vi "2-4_Ch Gen 0-20mA Current_9265.vi"() -> ()   [LabVIEW 2010]
doc: "I. Description:\nThis example demonstrates how to generate a single current value on one or more current output channels.\n\nII. Instructions for Running:\n1. Select the physical channel or channels which correspond to where your signal is to be generated.\n2. Enter the minimum and maximum current ranges, in amps (not milliamps).\n3. Enter a current value to generate in the data array. There should be one array value for each channel specified in the Physical Channels control. The values will be generated in the order that they appear in the Physical Channels control. \nNote: Just like the minimum and maximum current ranges, the data values to generate are in units of amps, not milliamps. \n\nIII. Block Diagram Steps:\n1. Create an analog output current channel.\n2. Call the Start VI to start the task.\n3. Use the Write VI to generate the data values on the\nspecified channels. Each element in the array contains\none current value for one channel specified in the \nPhysical Channels control.\n4. Call the Clear Task VI to clear the Task.\n5. Return any errors to the user in a dialog box.\n\nIV. I/O Connections Overview:\nThe SCXI-1124 can operate on either an external or internal current source. The only difference is in the signal connections. When using the internal current source, connect a load between the SUPPLY and ISINK terminals. When using an external current source, connect the source and load to the ISINK and GND terminals. In either case, be sure that the channel numbers of the terminals used match the channel numbers specified in the Physical Channels control.\n\nNote: When using an external current source, be careful to avoid creating an uncontrolled current loop. See the SCXI-1124 User's Manual for more information. \n\nThe NI 6238 and NI 6239 devices require external current sources. See the M Series User Manual for more information about signal connections to these devices.\n\nThe output current can be measured by connecting an ammeter in series with the current loop. Alternatively, the current can be measured by replacing the load with a resistor of known value. By measuring the voltage across the resistor and dividing by the resistance, the current through the resistor can be calculated (Ohm's law)."
uses:
  <vilib>/Utility/error.llb/DialogType.ctl
  <vilib>/Platform/TimedLoop/XDataNode/XDataNode.xnode
  <vilib>/Platform/TimedLoop/XDataNode/timing_clust.ctl
  <vilib>/Platform/TimedLoop/XDataNode/nitl_modes.ctl
  <vilib>/Platform/TimedLoop/XDataNode/wakeup.ctl
  <vilib>/DAQmx/write.llb/DAQmx Write (Analog 1D DBL NChan 1Samp).vi
  <vilib>/DAQmx/create/channels.llb/DAQmx Create Channel (AO-Current-Basic).vi
  <vilib>/daqmx/miscellaneous.llb/DAQmx Fill In Error Info.vi
  <vilib>/Analysis/NI_AALBase.lvlib
  <vilib>/Platform/TimedLoop/XDataNode/XDNodeRunTimeDep.lvlib
panel:
  out "transposed array":dbl[][](array[numeric]) format="%.4f"
  in  "Sine?":bool
  in  "Continuous?":bool
  in  "Apply":bool
  in  "stop":bool
  in  "Physical Channels":tag="cDAQ1Mod7/ao0:1"
  in  "Data":dbl[](array[slide])=[0.0, 0.0] min=0.0 max=0.02 step=0.001 scale=0.0..0.02 scale format="%.3f"
  in  "Minimum Value":dbl format="%0.3f"
  in  "Maximum Value":dbl=0.02 format="%0.3f"
  # "For instructions, select Help>>Show Context Help"
  # "Channel Parameters"
  # "Change to: \nao0:3 for 4-Ch\nMode, and add\nto array below."
  # "Current Values"
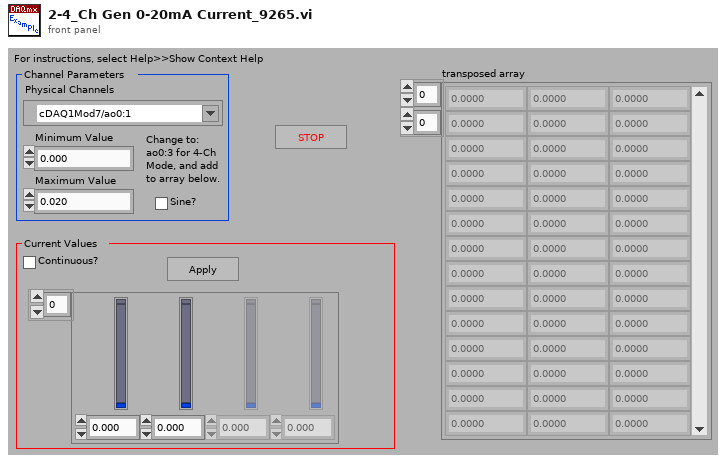
[diagram p1: front panel]
types:
  T1 = typedef "DialogType.ctl" = u16
  T2 = typedef "XDNodeRunTimeDep.lvlib/timing_clust.ctl" = cluster{"Expected End [f-1]":u64, "Actual End [f-1]":u64, "Finished Late? [f-1]":bool, "Expected End [i-1]":u64, "Actual End [i-1]":u64, "Finished Late? [i-1]":bool, "Expected Start [i]":u64, "Actual Start [i]":u64, "Expected Start [f]":u64, "Actual Start [f]":u64, "Source Name":string, "Structure Name":string, "Period":i64, "Deadline":i64, "Offset":i64, "Start":i64, "Priority":i32, "Timeout":i32, "Mode":T3, "Wakeup Reason":T4, "Error":errorcluster, "Source Type":string, "Secondary Source Type":string, "Global End Time":u64, "Global Start Time":u64, "Frame Duration":u64, "Iteration Duration":u64, "Assigned CPU":i32, "I/O Scan Engine Mode":u32}
  T3 = typedef "XDNodeRunTimeDep.lvlib/nitl_modes.ctl" = enum32{"No Change", "Process missed periods, maintain original phase", "Discard missed periods, maintain original phase", "Process missed periods, ignore original phase", "Discard missed periods, ignore original phase"}
  T4 = typedef "XDNodeRunTimeDep.lvlib/wakeup.ctl" = enum32{"Normal", "Aborted", "Asynchronous wakeup", "Timing source error", "Timed loop error", "Timeout"}
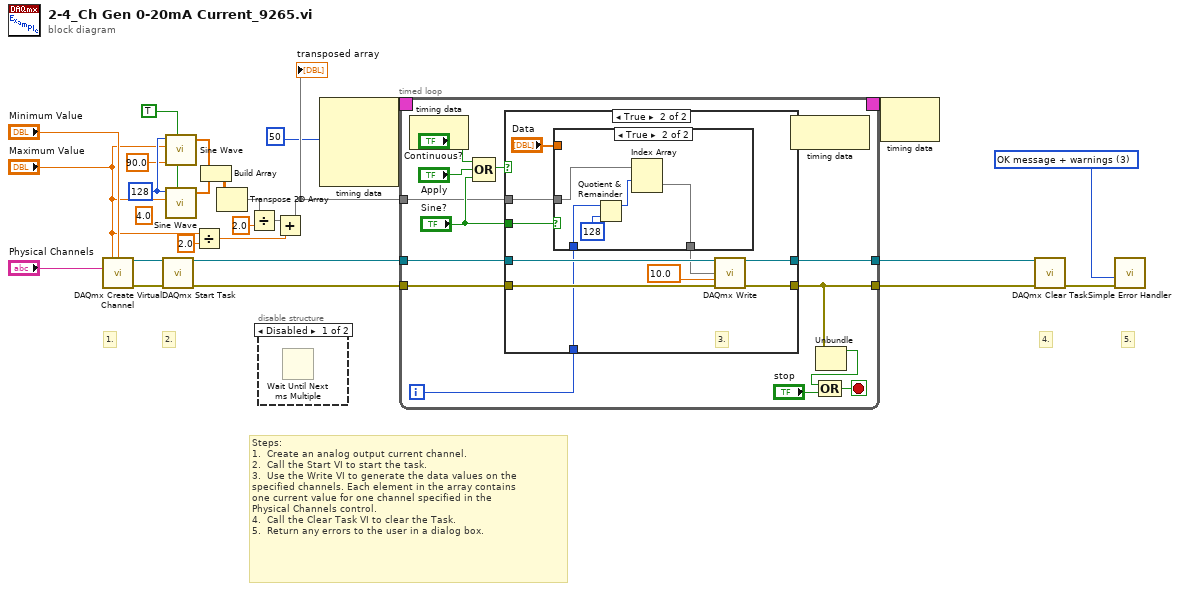
[diagram p0: block diagram]
diagram:
  w12 = TRUE ("reset phase")
  (unwired) 4.0 ("cycles")
  w16 = 128 ("samples")
  w19 = T1 3 items=["no dialog", "OK message", "continue or stop message", "OK message + warnings", "continue/stop + warnings"] ("type of dialog (OK msg:1)")
  # "5."
  # "Steps: \n1.  Create an analog output current channel.\n2.  Call the Start VI to start the task.\n3.  Use the Write VI to generate the data values on the\nspecified channels. Each element in the array contains\none current value for one channel specified in the \nPhysical Channels control.\n4.  Call the Clear Task VI to clear the Task.\n5.  Return any errors to the user in a dialog box."
  # "1."
  # "2."
  # "4."
  n1 = call-poly <vilib>:"DAQmx Create Virtual Channel.vi"("maximum value"="Maximum Value", "minimum value"="Minimum Value", "physical channels"="Physical Channels") -> ("task out"=w25:refnum<k21>, "error out"=w24:errorcluster)  [unwired: 11 in]
  n2 = call <vilib>:"DAQmx Start Task.vi"("task/channels in"=w25, "error in"=w24) -> ("task out"=w23:refnum<k21>, "error out"=w22:errorcluster)  [unwired: 12 in]
  n3 = call <vilib>:"Sine Wave.vi"("samples"=w16, "amplitude"="Maximum Value", "phase in"=90.0 ("phase(degrees)"), "reset phase"=w12) -> ("sine wave"=w15:dbl[])  [unwired: 1 in, 2 out]
  n4 = call <vilib>:"Sine Wave.vi"("samples"=w16, "amplitude"="Maximum Value", "reset phase"=w12) -> ("sine wave"=w14:dbl[])  [unwired: 2 in, 2 out]
  n5 = Divide(x="Maximum Value", y=2.0 ("cycles")) -> (x/y=w4:dbl)
  n6 = Build Array(w15, w14) -> (w13:dbl[][])
  n7 = Transpose 2D Array(2D array=w13) -> (transposed array=w10:dbl[][])
  n8 = Divide(x=w10, y=2.0 ("cycles")) -> (x/y=w8:dbl[][])
  n9 = disable-structure shown="Disabled" {
    frame Disabled {
      n10 = Wait Until Next ms Multiple() -> ()  [unwired: 1 in, 1 out]
    }
    frame Enabled {
    }
  }
  n11 = Add(x=w8, y=w4) -> (x+y=w7:dbl[][])
  "transposed array" <- w7
  n12 = node-c288(u32 50 ("millisecond multiple")) -> (w3:T2)  [unwired: 3 in]
  n13 = timed-loop {
    tunnel: w23 -> [w39]
    tunnel: w22 -> [w38]
    tunnel: [w37] -> w18
    tunnel: [w34] -> w17
    tunnel: w7 -> [w27]
    timing: w3 -> [_]
    timing-out: [_] -> w2
    i -> [w28]
    stop <- w35 stop-if-true
    n14 = node-c288() -> ()  [unwired: 1 in, 1 out]
    n15 = Compound Arithmetic op=OR("Continuous?", "Apply", "Sine?") -> (w30:bool)
    n16 = case shown="True" w30 {
      tunnel: w39 -> [w42 w53]
      tunnel: w38 -> [w43 w52]
      tunnel: [w42 w50] -> w37
      tunnel: [w43 w49] -> w34
      tunnel: "Sine?" -> [_ w46]
      tunnel: w28 -> [_ w45]
      tunnel: w27 -> [_ w44]
      frame False {
      }
      frame True {
        # "3."
        n17 = case shown="True" w46 {
          tunnel: "Data" -> [w54 _]
          tunnel: [w54 w55] -> w47
          tunnel: w45 -> [_ w59]
          tunnel: w44 -> [_ w56]
          frame False {
          }
          frame True {
            n18 = Quotient & Remainder(x=w59, y=128 ("samples")) -> (x-y*floor(x/y)=w57:i32)  [unwired: 1 out]
            n19 = Index Array(array=w56, index (row)=w57) -> (element=w55:dbl[])  [unwired: 1 in]
          }
        }
        n20 = call-poly <vilib>:"DAQmx Write.vi"("task/channels in"=w53, "data"=w47, "timeout"=10.0, "error in"=w52) -> ("task out"=w50:refnum<k21>, "error out"=w49:errorcluster)  [unwired: 9 in, 1 out]
      }
    }
    n21 = node-c288() -> ()  [unwired: 1 in, 1 out]
    n22 = Unbundle(w34) -> ("status"=w33:bool)  [unwired: 2 out]
    n23 = Compound Arithmetic op=OR(w33, "stop") -> (w35:bool)
  }
  n24 = node-c288(w2) -> ()  [unwired: 1 out]
  n25 = call <vilib>:"DAQmx Clear Task.vi"("task in"=w18, "error in"=w17) -> ("error out"=w21:errorcluster)  [unwired: 13 in]
  n26 = call <vilib>:"Simple Error Handler.vi"("type of dialog (OK msg:1)"=w19, "error in (no error)"=w21) -> ()  [unwired: 3 in, 5 out]
